vi "niRFUtil CONV Number to Bit Stream.vi"(0 "error in (no error)":errorcluster, 2 "Bit Stream In":T1 min=0, 3 "Number":u32 max=16777215 format="%.0x", 4 "Length":i32 max=32 format="%.0x") -> (1 "error out":errorcluster, 5 "Bit Stream Out":T1 min=0)   [LabVIEW 2015, in "niRFUtil.lvlib"]
uses:
  niRFUtil.lvlib
  Includes/niRFUtil INC Bit Array.ctl
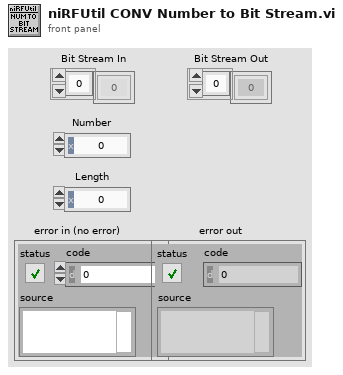
[diagram p1: front panel]
types:
  T1 = typedef "niRFUtil.lvlib/niRFUtil INC Bit Array.ctl" = i8[]
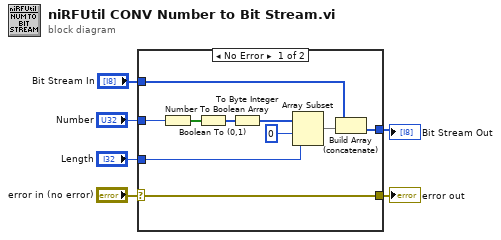
[diagram p0: block diagram]
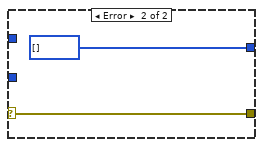
[diagram p2: hidden frame]
diagram:
  n1 = case shown="No Error" "error in (no error)" {
    selector: "error in (no error)" -> [w7 w17]
    tunnel: [w7 w17] -> w6
    tunnel: "Number" -> [w12 _]
    tunnel: [w10 i8[] [] ("Sync Word")] -> w4
    tunnel: "Length" -> [w11 _]
    tunnel: "Bit Stream In" -> [w8 _]
    frame No Error {
      n2 = Number To Boolean Array(number=w12) -> (Boolean array=w16:bool[])
      n3 = Boolean To (0,1)(Boolean=w16) -> (0, 1=w13:i16[])
      n4 = To Byte Integer(number=w13) -> (8bit integer=w14:i8[])
      n5 = Array Subset(array=w14, index=0, length=w11) -> (w9:i8[])
      n6 = Build Array (concatenate)(w8, w9) -> (w10:T1)
    }
    frame Error {
    }
  }
  "error out" <- w6
  "Bit Stream Out" <- w4
